vi "nanostage-coordinate-origin.vi"() -> ()   [LabVIEW 2015]
panel:
  out "picture number":u8 max=3 step=1
  in  "switch LR":bool
  out "Ring":u8(ring)
  in  "switch UD":bool
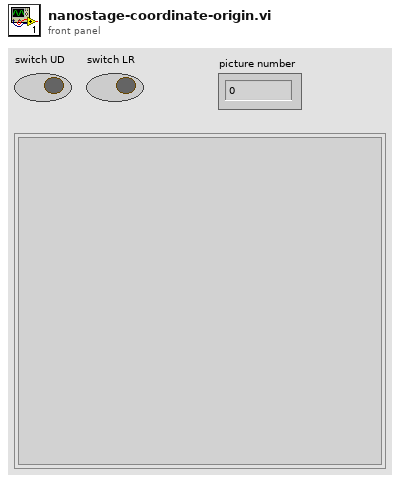
[diagram p1: front panel]
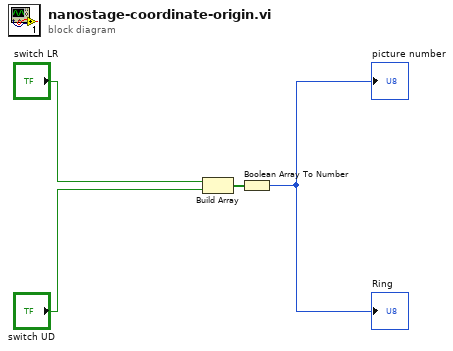
[diagram p0: block diagram]
diagram:
  n1 = Build Array("switch LR", "switch UD") -> (w4:bool[])
  n2 = Boolean Array To Number(Boolean array=w4) -> (number=→"Ring" →"picture number":u32)
